vi "panel.vi"() -> ()   [LabVIEW 2014]
uses:
  <vilib>/Utility/inputDevices.llb/mouseAcquire.vi
  <vilib>/Utility/inputDevices.llb/keyboardAcquire.vi
panel:
  out "r":i16
  out "angle":i16
  in  "Boolean":bool
  out "XY Graph":cluster{dbl[], dbl[]}(graph)
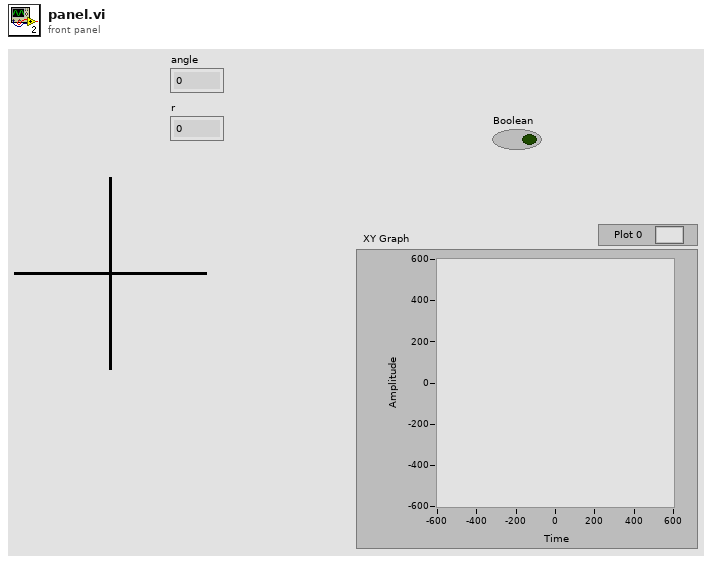
[diagram p1: front panel]
types:
  T1 = enum16{"0", "1", "2", "3", "4", "5", "6", "7", "8", "9", "A", "B", "C", "D", "E", "F", "G", "H", "I", "J", "K", "L", "M", "N", "O", "P", "Q", "R", "S", "T", "U", "V", "W", "X", "Y", "Z", "F1", "F2", "F3", "F4", "F5", "F6", "F7", "F8", "F9", "F10", "F11", "F12", "F13", "F14", "F15", "ADD", "BACK", "BACKSLASH", "CAPITAL", "COMMA", "DECIMAL", "DELETE", "DIVIDE", "DOWN", "END", "EQUALS", "ESCAPE", "GRAVE (`)", "HOME", "INSERT", "LBRACKET", "LCONTROL", "LEFT", "L ALT", "LSHIFT", "LWIN", "MINUS", "MULTIPLY", "NEXT", "NUMLOCK", "NUMPAD_0", "NUMPAD_1", "NUMPAD_2", "NUMPAD_3", "NUMPAD_4", "NUMPAD_5", "NUMPAD_6", "NUMPAD_7", "NUMPAD_8", "NUMPAD_9", "PAUSE", "PERIOD", "PRIOR (PG UP)", "RBRACKET", "RCONTROL", "RETURN", "RIGHT", "R ALT", "RSHIFT", "RWIN", "SCROLL", "SEMICOLON", "SLASH", "SPACE", "SUBTRACT", "TAB", "UP", "ENTER (num pad)", "' (quote)"}[][]
  T2 = typedef "LVRectTypeDef.ctl" = cluster{"Left":i16, "Top":i16, "Right":i16, "Bottom":i16}
  T3 = typedef "LVPointTypeDef.ctl" = cluster{"Horizontal":i16, "Vertical":i16}
  T4 = cluster{"Horizontal":i32, "Vertical":i32, "Scrolling":i32}
  T5 = cluster{"button 1":bool, "button 2":bool, "button 3":bool, "button 4":bool}
  T6 = enum16{"0", "1", "2", "3", "4", "5", "6", "7", "8", "9", "A", "B", "C", "D", "E", "F", "G", "H", "I", "J", "K", "L", "M", "N", "O", "P", "Q", "R", "S", "T", "U", "V", "W", "X", "Y", "Z", "F1", "F2", "F3", "F4", "F5", "F6", "F7", "F8", "F9", "F10", "F11", "F12", "F13", "F14", "F15", "ADD", "BACK", "BACKSLASH", "CAPITAL", "COMMA", "DECIMAL", "DELETE", "DIVIDE", "DOWN", "END", "EQUALS", "ESCAPE", "GRAVE (`)", "HOME", "INSERT", "LBRACKET", "LCONTROL", "LEFT", "L ALT", "LSHIFT", "LWIN", "MINUS", "MULTIPLY", "NEXT", "NUMLOCK", "NUMPAD_0", "NUMPAD_1", "NUMPAD_2", "NUMPAD_3", "NUMPAD_4", "NUMPAD_5", "NUMPAD_6", "NUMPAD_7", "NUMPAD_8", "NUMPAD_9", "PAUSE", "PERIOD", "PRIOR (PG UP)", "RBRACKET", "RCONTROL", "RETURN", "RIGHT", "R ALT", "RSHIFT", "RWIN", "SCROLL", "SEMICOLON", "SLASH", "SPACE", "SUBTRACT", "TAB", "UP", "ENTER (num pad)", "' (quote)"}[]
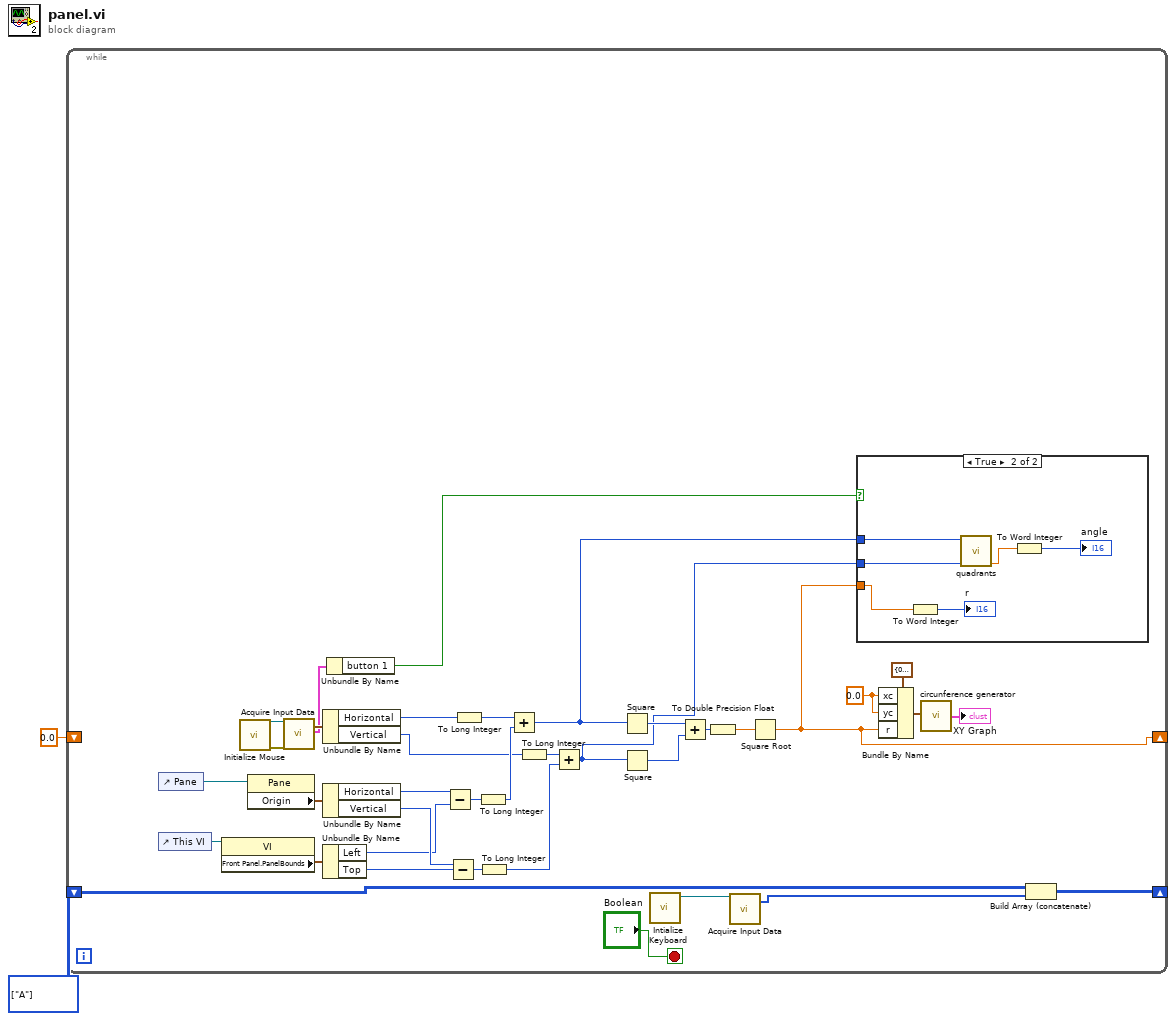
[diagram p0: block diagram]
diagram:
  w1 = T1 [[enum."A"]] items=["0", "1", "2", "3", "4", "5", "6", "7", "8", "9", "A", "B", "C", "D", "E", "F", "G", "H", "I", "J", "K", "L", "M", "N", "O", "P", "Q", "R", "S", "T", "U", "V", "W", "X", "Y", "Z", "F1", "F2", "F3", "F4", "F5", "F6", "F7", "F8", "F9", "F10", "F11", "F12", "F13", "F14", "F15", "ADD", "BACK", "BACKSLASH", "CAPITAL", "COMMA", "DECIMAL", "DELETE", "DIVIDE", "DOWN", "END", "EQUALS", "ESCAPE", "GRAVE (`)", "HOME", "INSERT", "LBRACKET", "LCONTROL", "LEFT", "L ALT", "LSHIFT", "LWIN", "MINUS", "MULTIPLY", "NEXT", "NUMLOCK", "NUMPAD_0", "NUMPAD_1", "NUMPAD_2", "NUMPAD_3", "NUMPAD_4", "NUMPAD_5", "NUMPAD_6", "NUMPAD_7", "NUMPAD_8", "NUMPAD_9", "PAUSE", "PERIOD", "PRIOR (PG UP)", "RBRACKET", "RCONTROL", "RETURN", "RIGHT", "R ALT", "RSHIFT", "RWIN", "SCROLL", "SEMICOLON", "SLASH", "SPACE", "SUBTRACT", "TAB", "UP", "ENTER (num pad)", "' (quote)"] ("Array")
  n1 = while {
    shift-right: [w3] -> _
    shift-left: 0.0 -> [_]
    shift-right: [w14] -> _
    shift-left: w1 -> [w15]
    stop <- "Boolean" stop-if-true
    w9 = 0.0 ("xc")
    n2 = control-ref of="Pane"() -> (w36:refnum<vi>)
    n3 = control-ref of="This VI"() -> (w34:refnum<vi>)
    n4 = property class="VI"(reference=w34) -> ("Front Panel.PanelBounds"=w33:T2)  [unwired: 1 in, 2 out]
    n5 = call <vilib>:"Initialize Mouse.vi"() -> ("error out"=w38:errorcluster, "device ID"=w39:refnum<k1>)  [unwired: 10 in]
    n6 = property class="Pane"(reference=w36) -> ("Origin"=w35:T3)  [unwired: 1 in, 2 out]
    n7 = call-poly <vilib>:"Acquire Input Data.vi"("device ID"=w39, "error in (no error)"=w38) -> ("axis info"=w37:T4, "button info"=w17:T5)  [unwired: 14 in, 2 out]
    n8 = Unbundle By Name(w37) -> ("Horizontal"=w30:i32, "Vertical"=w23:i32)
    n9 = Unbundle By Name(w35) -> ("Horizontal"=w29:i16, "Vertical"=w27:i16)
    n10 = Unbundle By Name(w33) -> ("Left"=w26:i16, "Top"=w28:i16)
    n11 = Unbundle By Name(w17) -> ("button 1"=w4:bool)
    n12 = Subtract(x=w29, y=w26) -> (x-y=w32:i16)
    n13 = Subtract(x=w27, y=w28) -> (x-y=w31:i16)
    n14 = To Long Integer(number=w30) -> (32bit integer=w22:i32)
    n15 = To Long Integer(number=w32) -> (32bit integer=w25:i32)
    n16 = To Long Integer(number=w31) -> (32bit integer=w24:i32)
    n17 = Add(x=w22, y=w25) -> (x+y=w6:i32)
    n18 = To Long Integer(number=w23) -> (32bit integer=w21:i32)
    n19 = Add(x=w21, y=w24) -> (x+y=w5:i32)
    n20 = Square(x=w6) -> (x^2=w8:i32)
    n21 = Square(x=w5) -> (x^2=w7:i32)
    n22 = call <vilib>:"Intialize Keyboard.vi"() -> ("device ID"=w16:refnum<k1>)  [unwired: 10 in, 1 out]
    n23 = Add(x=w8, y=w7) -> (x+y=w19:i32)
    n24 = To Double Precision Float(number=w19) -> (double precision float=w18:dbl)
    n25 = call-poly <vilib>:"Acquire Input Data.vi"("device ID"=w16) -> ("keys pressed"=w13:T6)  [unwired: 16 in, 2 out]
    n26 = Square Root(x=w18) -> (sqrt(x)=w3:dbl)
    n27 = case shown="True" w4 {
      tunnel: w6 -> [_ w44]
      tunnel: w5 -> [_ w43]
      tunnel: w3 -> [_ w42]
      frame False {
      }
      frame True {
        n28 = To Word Integer(number=w42) -> (16bit integer=→"r":i16)
        n29 = call "quadrants.vi"("y"=w43, "x"=w44) -> ("angle"=w45:dbl)  [unwired: 9 in]
        n30 = To Word Integer(number=w45) -> (16bit integer=→"angle":i16)
      }
    }
    n31 = Bundle By Name(cluster=cluster{"xc":dbl, "yc":dbl, "r":dbl} {"xc"=0.0, "yc"=0.0, "r"=0.0} ("input"), "xc"=w9, "yc"=w9, "r"=w3) -> (w11:cluster{"xc":dbl, "yc":dbl, "r":dbl})
    n32 = call "circunference generator.vi"("input"=w11) -> ("graph"=→"XY Graph":cluster{dbl[], dbl[]})  [unwired: 4 in]
    n33 = Build Array (concatenate)(w15, w13) -> (w14:T1)
  }
